vi "query Number Of Autodetected Cyclones.vi"(8 "error in":errorcluster) -> (0 "error out":errorcluster, 3 "function return":u32)   [LabVIEW 2021, in "CycloneControlSDK.lvlib"]
doc: "extern \"C\" uint32_t _cdecl queryNumberOfAutodetectedCyclones(void);"
uses:
  CycloneControlSDK.lvlib
  CycloneControlSDK_64.dll
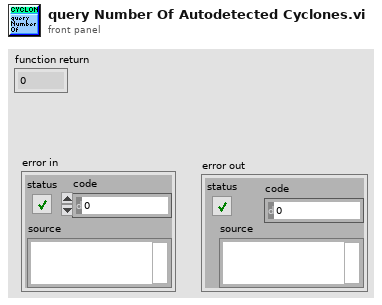
[diagram p1: front panel]
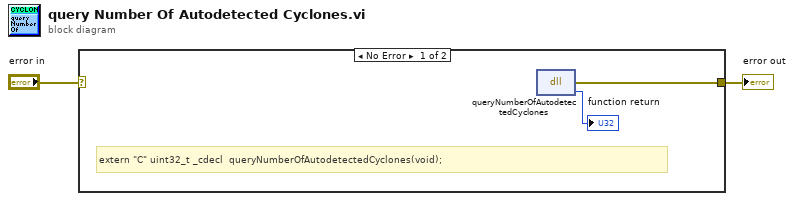
[diagram p0: block diagram]
diagram:
  n1 = case shown="No Error" "error in" {
    selector: "error in" -> [_ w5]
    tunnel: [w3 w5] -> w1
    frame No Error {
      # "extern \"C\" uint32_t _cdecl  queryNumberOfAutodetectedCyclones(void);"
      n2 = dll-call lib="C:/PEMicro/cyclone/cycloneControl/controlsdk/examples/labview2018/user.lib/CycloneControlSDK/CycloneControlSDK_64.dll" fn="queryNumberOfAutodetectedCyclones"() -> (error out=w3:errorcluster, "return type"=→"function return":u32)  [unwired: 3 in, 1 out]
    }
    frame Error {
    }
  }
  "error out" <- w1
